vi "Deform_Mirror_AbberationList_ae.vi"(0 "Mirror ID":string, 1 "Enum":enum16{"WRITE", "READ"}(ring), 11 "Abberation Cluster In":T1) -> (4 "Mirror ID Out":string, 15 "Abberation Cluster Out":T1)   [LabVIEW 2015]
uses:
  AbberationControl.ctl
panel:
  in  "Mirror ID":cluster{"Top":T1, "Bottom":T1}
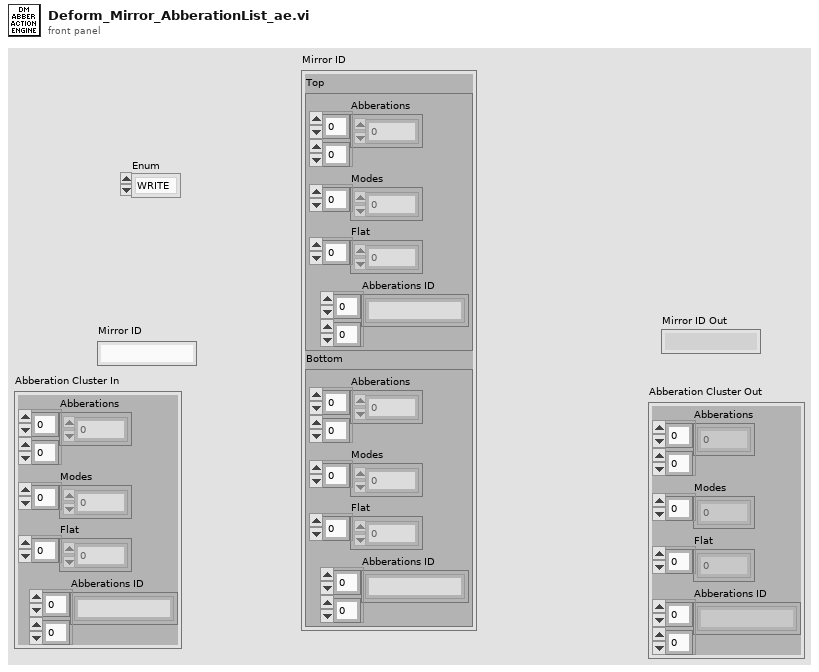
[diagram p1: front panel]
types:
  T1 = typedef "AbberationControl.ctl" = cluster{"Abberations":dbl[][], "Modes":i32[], "Flat":dbl[], "Abberations ID":string[][]}
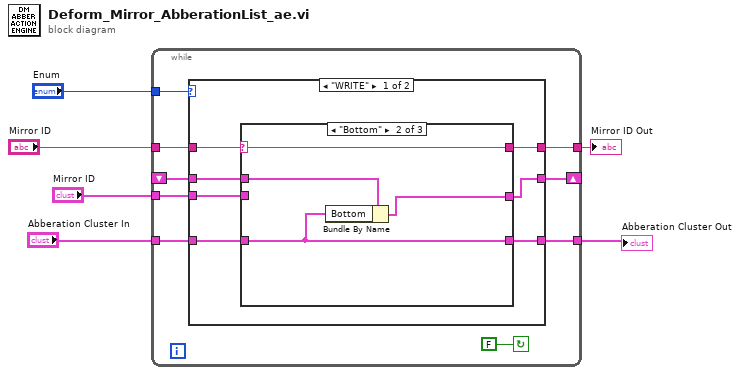
[diagram p0: block diagram]
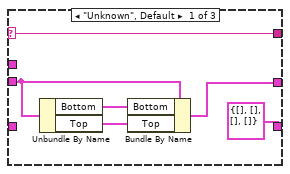
[diagram p2: hidden frame]
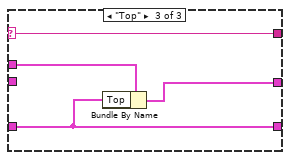
[diagram p3: hidden frame]
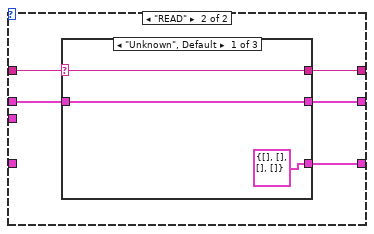
[diagram p4: hidden frame]
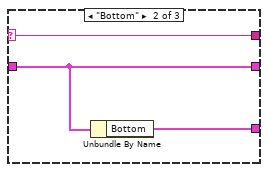
[diagram p5: hidden frame]
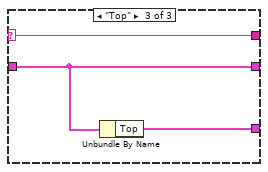
[diagram p6: hidden frame]
diagram:
  n1 = while {
    tunnel: "Enum" -> [w14]
    tunnel: "Abberation Cluster In" -> [w13]
    tunnel: "Mirror ID" -> [w12]
    shift-right: [w10] -> _
    shift-left: _ -> [w8]
    tunnel: "Mirror ID" -> [w11]
    tunnel: [w9] -> w2
    tunnel: [w7] -> w1
    stop <- FALSE continue-if-true
    n2 = case shown="\"WRITE\"" w14 {
      tunnel: w13 -> [w20 _]
      tunnel: w12 -> [w22 w41]
      tunnel: w11 -> [w21 _]
      tunnel: [w19 w40] -> w10
      tunnel: [w18 w38] -> w9
      tunnel: w8 -> [w17 w39]
      tunnel: [w16 w37] -> w7
      frame "WRITE" {
        n3 = case shown="\"Bottom\"" w22 {
          selector: w22 -> [w23 w29 w33]
          tunnel: w21 -> [w25 _ _]
          tunnel: w20 -> [_ w31 w35]
          tunnel: [w28 w32 w36] -> w19
          tunnel: [T1 {"Abberations"=[], "Modes"=[], "Flat"=[], "Abberations ID"=[]} ("Abberation Cluster In") w31 w35] -> w18
          tunnel: w17 -> [_ w30 w34]
          tunnel: [w23 w29 w33] -> w16
          frame "Unknown", Default {
            n4 = Unbundle By Name(w25) -> ("Bottom"=w27:T1, "Top"=w26:T1)
            n5 = Bundle By Name(cluster=w25, "Bottom"=w27, "Top"=w26) -> (w28:cluster{"Top":T1, "Bottom":T1})
          }
          frame "Bottom" {
            n6 = Bundle By Name(cluster=w30, "Bottom"=w31) -> (w32:cluster{"Top":T1, "Bottom":T1})
          }
          frame "Top" {
            n7 = Bundle By Name(cluster=w34, "Top"=w35) -> (w36:cluster{"Top":T1, "Bottom":T1})
          }
        }
      }
      frame "READ" {
        n8 = case shown="\"Unknown\", Default" w41 {
          selector: w41 -> [w42 w45 w48]
          tunnel: [w44 w47 w50] -> w40
          tunnel: w39 -> [w44 w47 w50]
          tunnel: [T1 {"Abberations"=[], "Modes"=[], "Flat"=[], "Abberations ID"=[]} ("Top") w46 w49] -> w38
          tunnel: [w42 w45 w48] -> w37
          frame "Unknown", Default {
          }
          frame "Bottom" {
            n9 = Unbundle By Name(w47) -> ("Bottom"=w46:T1)
          }
          frame "Top" {
            n10 = Unbundle By Name(w50) -> ("Top"=w49:T1)
          }
        }
      }
    }
  }
  "Abberation Cluster Out" <- w2
  "Mirror ID Out" <- w1
